vi "PicoReleaseMultiBuffers.vi"(8 "error in (no error)":errorcluster, 9 "Enabled array":i16[](array[numeric]), 10 "Data Pointers":T1) -> (0 "error out":errorcluster)   [LabVIEW 2020]
doc: "Release Picodata buffers for Block and 6000a streaming examples"
uses:
  PicoBuffers.ctl
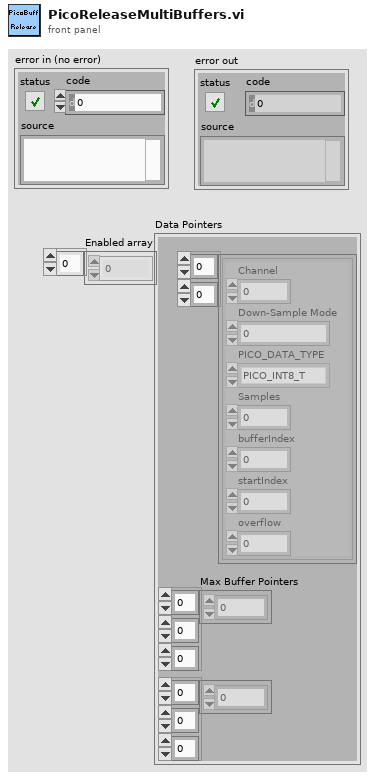
[diagram p1: front panel]
types:
  T1 = typedef "PicoBuffers.ctl" = cluster{"Max Buffer Pointers":u64[][][], "Min Buffer Pointers":u64[][][], "StreamingDataInfo":cluster{"Channel":u32, "Down-Sample Mode":u32, "PICO_DATA_TYPE":enum32{"PICO_INT8_T", "PICO_INT16_T", "PICO_INT32_T", "PICO_UINT32_T", "PICO_INT64_T", ""}, "Samples":i32, "bufferIndex":u64, "startIndex":i32, "overflow":i16}[][]}
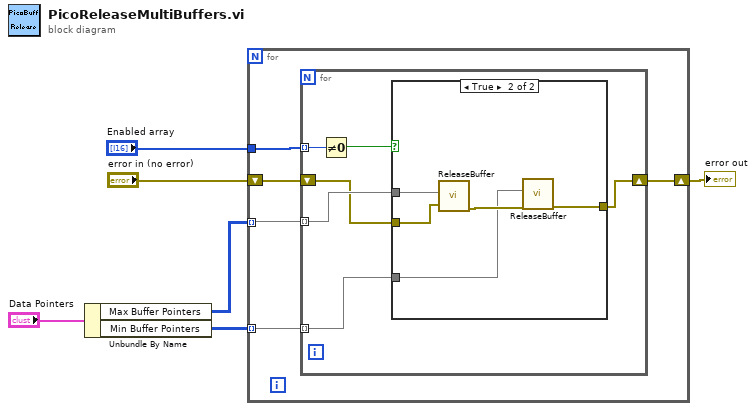
[diagram p0: block diagram]
diagram:
  n1 = Unbundle By Name("Data Pointers") -> ("Max Buffer Pointers"=w2:u64[][][], "Min Buffer Pointers"=w1:u64[][][])
  n2 = for {
    tunnel: w2 -> [w11] mode=indexing
    shift-right: [w9] -> w5
    shift-left: "error in (no error)" -> [w10]
    tunnel: "Enabled array" -> [w8]
    tunnel: w1 -> [w7] mode=indexing
    n3 = for {
      tunnel: w11 -> [w17] mode=indexing
      tunnel: w8 -> [w16] mode=indexing
      shift-right: [w14] -> w9
      shift-left: w10 -> [w15]
      tunnel: w7 -> [w13] mode=indexing
      n4 = Not Equal To 0?(x=w16) -> (x != 0?=w12:bool)
      n5 = case shown="True" w12 {
        tunnel: w17 -> [_ w23]
        tunnel: w15 -> [w18 w22]
        tunnel: [w18 w20] -> w14
        tunnel: w13 -> [_ w19]
        frame False {
        }
        frame True {
          n6 = call "ReleaseBuffer.vi"("error in (no error)"=w22, "Pointer and BufferSize"=w23) -> ("error out"=w21:errorcluster)  [unwired: 9 in]
          n7 = call "ReleaseBuffer.vi"("error in (no error)"=w21, "Pointer and BufferSize"=w19) -> ("error out"=w20:errorcluster)  [unwired: 9 in]
        }
      }
    }
  }
  "error out" <- w5
